vi "Test.vi"() -> ()   [LabVIEW 2014]
uses:
  C:/Users/iknox/Documents/Visual Studio 2013/Projects/ConvertListToArray/ConvertListToArray/ClassLibrary1/bin/Debug/ListToArrayWrapper.dll
  Users/iknox/Documents/Visual Studio 2013/Projects/ConvertListToArray/ConvertListToArray/ClassLibrary1/bin/Debug/ListToArrayWrapper.dll
  Microsoft.Kinect
  controls/BodyData.ctl
panel:
  out "Body Data":T1[](array[typedef]) {"LeanTrackingState" items=["NotTracked", "Inferred", "Tracked"]; "HandRightState" items=["Unknown", "NotTracked", "Open", "Closed", "Lasso"]; "HandRightConfidence" items=["Low", "High"]; "HandLeftState" items=["Unknown", "NotTracked", "Open", "Closed", "Lasso"]; "HandLeftConfidence" items=["Low", "High"]; "ClippedEdges" items=["None"=0, "Right"=1, "Left"=2, "Top"=4, "Bottom"=8]}
  in  "Enabled Frames":T2={"Color"=TRUE, "Infrared"=FALSE, "LongExposureInfrared"=FALSE, "Depth"=FALSE, "BodyIndex"=FALSE, "Body"=FALSE, "Audio"=FALSE}
  in  "stop":bool
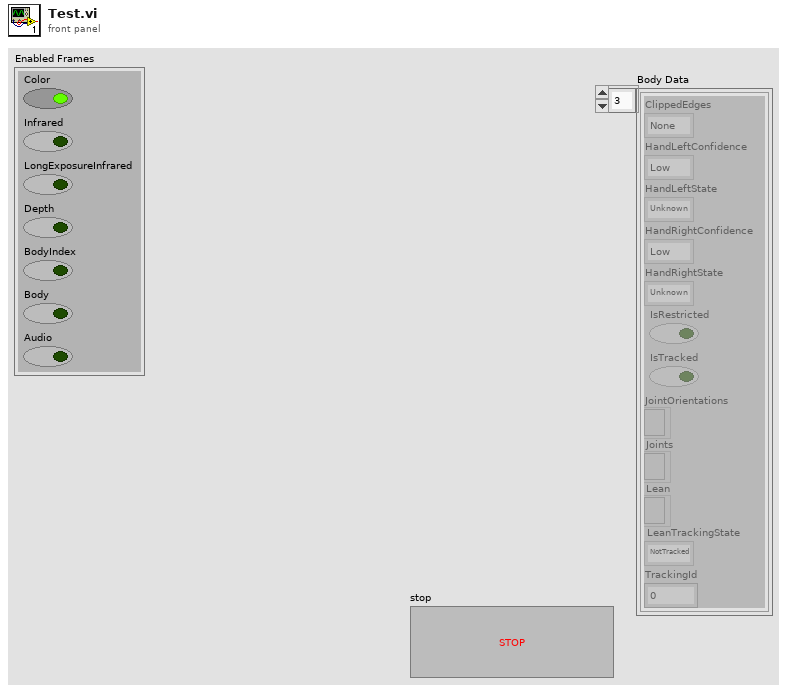
[diagram p1: front panel]
types:
  T1 = typedef "BodyData.ctl" = cluster{"ClippedEdges":i32, "HandLeftConfidence":i32, "HandLeftState":i32, "HandRightConfidence":i32, "HandRightState":i32, "IsRestricted":bool, "IsTracked":bool, "JointOrientations":refnum<k24>, "Joints":refnum<k24>, "Lean":refnum<k24>, "LeanTrackingState":i32, "TrackingId":u64}
  T2 = cluster{"Color":bool, "Infrared":bool, "LongExposureInfrared":bool, "Depth":bool, "BodyIndex":bool, "Body":bool, "Audio":bool}
  T3 = typedef "KinectSensor References.ctl" = cluster{"KinectSensorRefnum":refnum<k24>, "MultiSourceFrameReader":refnum<k24>}
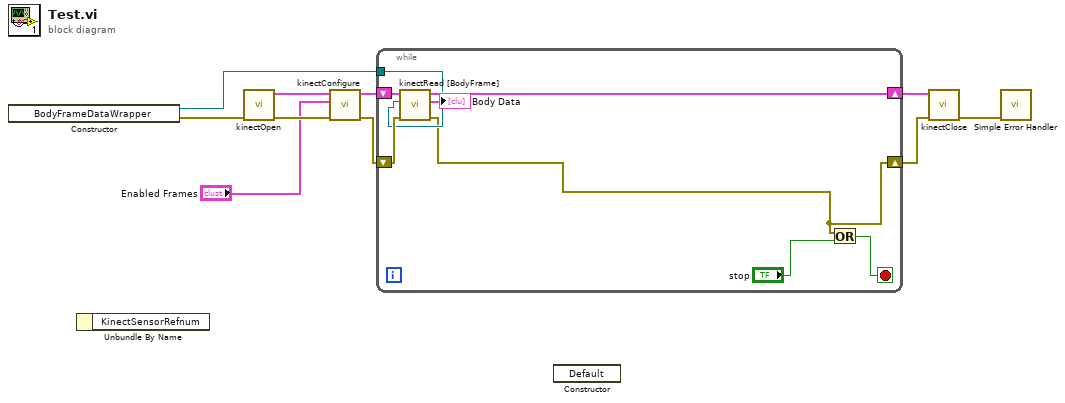
[diagram p0: block diagram]
diagram:
  n1 = constructor class="BodyFrameDataWrapper"() -> (reference out=w1:refnum<k24>, error out=w2:errorcluster)  [unwired: 3 in, 1 out]
  n2 = Unbundle By Name() -> ()  [unwired: 1 in, 1 out]
  n3 = call "kinectOpen.vi"("error in (no error)"=w2) -> ("error out"=w10:errorcluster, "KinectSensor References"=w8:T3)  [unwired: 9 in]
  n4 = call "kinectConfigure.vi"("error in (no error)"=w10, "Enabled Frames"="Enabled Frames", "KinectSensor References in"=w8) -> ("error out"=w9:errorcluster, "KinectSensor References out"=w6:T3)  [unwired: 7 in]
  n5 = while {
    shift-right: [w12] -> w4
    shift-left: w9 -> [w14]
    shift-right: [w15] -> w5
    shift-left: w6 -> [w16]
    tunnel: w1 -> [w13]
    stop <- w17 stop-if-true
    n6 = call "kinectRead [BodyFrame].vi"("error in (no error)"=w14, "Wrapper Reference"=w13, "KinectSensor References in"=w16) -> ("error out"=w12:errorcluster, "Body Data"=→"Body Data":T1[], "KinectSensor References out"=w15:T3)  [unwired: 6 in]
    n7 = Or(x=w12, y="stop") -> (x .or. y?=w17:bool)
  }
  n8 = constructor class=".NET"() -> ()  [unwired: 3 in, 3 out]
  n9 = call "kinectClose.vi"("error in"=w4, "KinectSensor References"=w5) -> ("error out"=w3:errorcluster)  [unwired: 9 in]
  n10 = call <vilib>:"Simple Error Handler.vi"("error in (no error)"=w3) -> ()  [unwired: 4 in, 5 out]
